vi "value to ring (FilterMode).vi"(11 "value":string) -> (3 "FilterMode":u32)   [LabVIEW 2020, in "AIM ARINC 664 Import.lvlib"]
uses:
  AIM ARINC 664 Import.lvlib
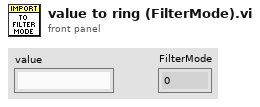
[diagram p1: front panel]
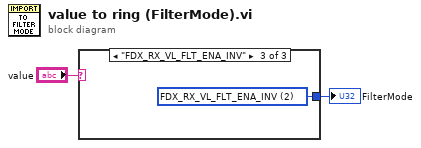
[diagram p0: block diagram]
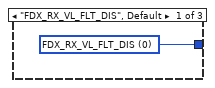
[diagram p2: hidden frame]
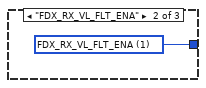
[diagram p3: hidden frame]
diagram:
  n1 = case shown="\"FDX_RX_VL_FLT_ENA_INV\"" "value" {
    tunnel: [w3 w4 w5] -> w1
    frame "FDX_RX_VL_FLT_DIS", Default {
      w3 = u32 0 items=["FDX_RX_VL_FLT_DIS", "FDX_RX_VL_FLT_ENA ", "FDX_RX_VL_FLT_ENA_INV"] ("FilterMode")
    }
    frame "FDX_RX_VL_FLT_ENA" {
      w4 = u32 1 items=["FDX_RX_VL_FLT_DIS", "FDX_RX_VL_FLT_ENA ", "FDX_RX_VL_FLT_ENA_INV"] ("FilterMode")
    }
    frame "FDX_RX_VL_FLT_ENA_INV" {
      w5 = u32 2 items=["FDX_RX_VL_FLT_DIS", "FDX_RX_VL_FLT_ENA ", "FDX_RX_VL_FLT_ENA_INV"] ("FilterMode")
    }
  }
  "FilterMode" <- w1
